vi "01-Init and Load Project.vi"() -> ()   [LabVIEW 2022 SP3, in "LV_VGS.lvlib"]
uses:
  LV_VGS.lvlib
  RemoteControlClient/VGS_RemoteControlClient.lvclass
panel:
  in  "path":path=path "C:/Program Files/Volume Graphics/VGStudio MAX 22/Data/01-FirstSteps.vgl"
  out "LastWarning":string
  out "LastError 2":string
  out "LastError":string
  out "Numeric":i32
  in  "stop":bool
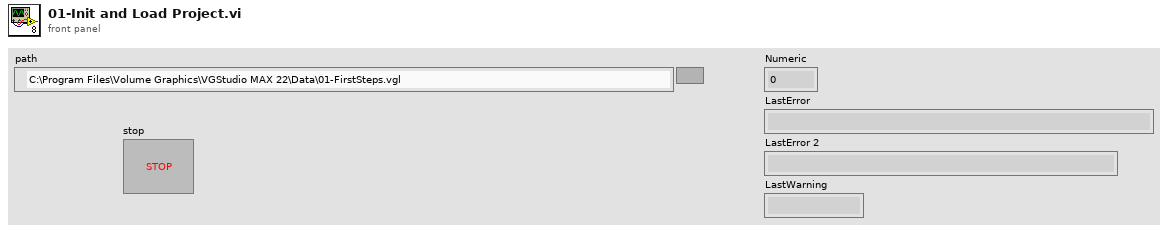
[diagram p1: front panel]
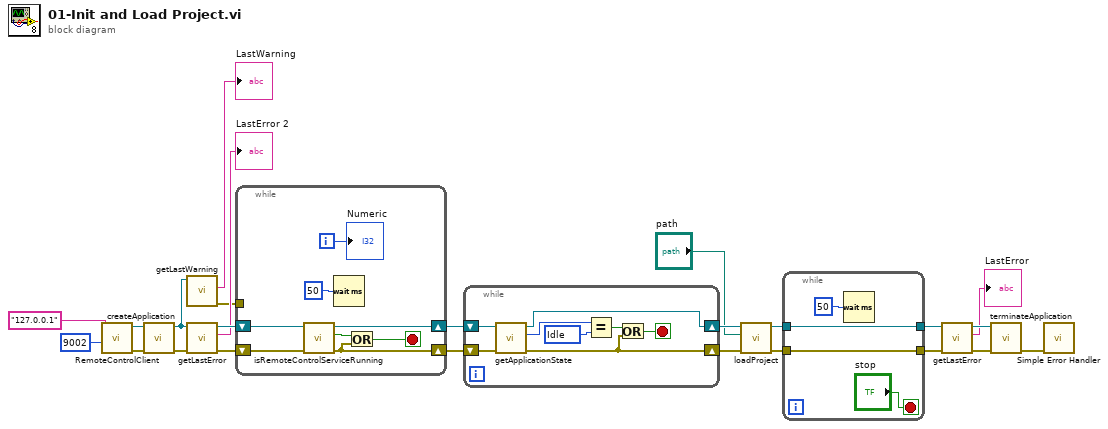
[diagram p0: block diagram]
diagram:
  n1 = call "RemoteControlClient.vi"("servicePort (9002)"=9002, "(localhost)"="127.0.0.1") -> ("error out"=w23:errorcluster, "VGS_RemoteControlClient out"=w24:refnum<class "VGS_RemoteControlClient.lvclass">)  [unwired: 8 in]
  n2 = call "createApplication.vi"("error in (no error)"=w23, "VGS_RemoteControlClient in"=w24) -> ("error out"=w14:errorcluster, "VGS_RemoteControlClient out"=w11:refnum<class "VGS_RemoteControlClient.lvclass">)  [unwired: 8 in]
  n3 = call "getLastWarning.vi"("VGS_RemoteControlClient in"=w11) -> ("error out"=w10:errorcluster, "LastWarning"=→"LastWarning":string)  [unwired: 8 in, 1 out]
  n4 = call "getLastError.vi"("error in (no error)"=w14, "VGS_RemoteControlClient in"=w11) -> ("error out"=w13:errorcluster, "LastError"=→"LastError 2":string, "VGS_RemoteControlClient out"=w15:refnum<class "VGS_RemoteControlClient.lvclass">)  [unwired: 7 in]
  n5 = while {
    shift-right: [w29] -> w6
    shift-left: w15 -> [w32]
    shift-right: [w25] -> w5
    shift-left: w13 -> [w28]
    tunnel: w10 -> [_]
    i -> [w27]
    stop <- w26 stop-if-true
    n6 = call "isRemoteControlServiceRunning.vi"("error in (no error)"=w28, "VGS_RemoteControlClient in"=w32) -> ("error out"=w25:errorcluster, "isRemoteControlServiceRunning"=w31:bool, "VGS_RemoteControlClient out"=w29:refnum<class "VGS_RemoteControlClient.lvclass">)  [unwired: 7 in]
    n7 = Wait (ms)(milliseconds to wait=u32 50) -> ()  [unwired: 1 out]
    n8 = Or(x=w31, y=w25) -> (x .or. y?=w26:bool)
    "Numeric" <- w27
  }
  n9 = while {
    shift-right: [w37] -> w3
    shift-left: w6 -> [w40]
    shift-right: [w33] -> w4
    shift-left: w5 -> [w36]
    stop <- w34 stop-if-true
    w38 = 1448165379 items=["NotRunning"=1448165376, "Starting"=1448165377, "Dying"=1448165378, "Idle"=1448165379, "WorkInProgress"=1448165380] ("getApplicationState")
    n10 = call "getApplicationState.vi"("error in (no error)"=w36, "VGS_RemoteControlClient in"=w40) -> ("error out"=w33:errorcluster, "getApplicationState"=w39:i32, "VGS_RemoteControlClient out"=w37:refnum<class "VGS_RemoteControlClient.lvclass">)  [unwired: 7 in]
    n11 = Equal?(x=w39, y=w38) -> (x = y?=w35:bool)
    n12 = Or(x=w35, y=w33) -> (x .or. y?=w34:bool)
  }
  n13 = call "loadProject.vi"("error in (no error)"=w4, "projectName"="path", "VGS_RemoteControlClient in"=w3) -> ("error out"=w8:errorcluster, "VGS_RemoteControlClient out"=w7:refnum<class "VGS_RemoteControlClient.lvclass">)  [unwired: 7 in]
  n14 = while {
    tunnel: w7 -> [w42]
    tunnel: [w42] -> w19
    tunnel: [w41] -> w20
    tunnel: w8 -> [w41]
    stop <- "stop" stop-if-true
    n15 = Wait (ms)(milliseconds to wait=u32 50) -> ()  [unwired: 1 out]
  }
  n16 = call "getLastError.vi"("error in (no error)"=w20, "VGS_RemoteControlClient in"=w19) -> ("error out"=w16:errorcluster, "LastError"=→"LastError":string, "VGS_RemoteControlClient out"=w18:refnum<class "VGS_RemoteControlClient.lvclass">)  [unwired: 7 in]
  n17 = call "terminateApplication.vi"("error in (no error)"=w16, "VGS_RemoteControlClient in"=w18) -> ("error out"=w22:errorcluster)  [unwired: 8 in, 1 out]
  n18 = call <vilib>:"Simple Error Handler.vi"("error in (no error)"=w22) -> ()  [unwired: 4 in, 5 out]
